vi "Compute Magnitudes.vi"(5 "view mode":enum16{"Power", "Amplitude", "dB"}(ring)=enum."Amplitude", 6 "averaging parameters":T1={"exponential mode"=enum."Fast", "time constant [ms]"=125.0, "decimating factor"=1} {"decimating factor" min=1 step=1; "time constant [ms]" format="%.2f"}, 7 "rpm range (auto)":T3 {"increment" format="%.2f"; "maximum" format="%.2f"; "minimum" format="%.2f"}, 9 "averaging type":enum16{"Linear", "Exponential"}(ring), 10 "speed profile":T4 {"speed [RPM]" format="%.2f"; "time [s]" format="%.2f"}, 11 "order waveforms [EU]":waveform(dbl)[](array[waveform])) -> (1 "unit label":string, 2 "magnitudes vs. rpm":T2(array[cluster]) {"magnitude" format="%.2f"; "delta rpm" format="%.2f"; "rpm 0" format="%.2f"}, 3 "orders magnitudes":waveform(dbl)[](array[waveform]))   [LabVIEW 2017]
doc: "Computes magnitudes for the order time waveforms."
uses:
  <vilib>/addons/Sound and Vibration/Order Analysis/Tach Process/SubVIs/speed profile.ctl
  <vilib>/addons/_NISVFA/_Shared subVIs/Common/svc_Engineering Units to Unit Label.vi
  <vilib>/addons/_NISVFA/_Shared subVIs/Common/svc_Unit Label to Engineering Units.vi
  <vilib>/Waveform/WDTOps.llb/WDT Index Channel DBL.vi
  <vilib>/addons/Sound and Vibration/Order Analysis/Gabor Order Tracking/SoundVib_Gabor.lvlib
  <vilib>/addons/Sound and Vibration/Order Analysis/Tach Process/SoundVib_TachProcess.lvlib
panel:
  # "Compute Magnitudes"
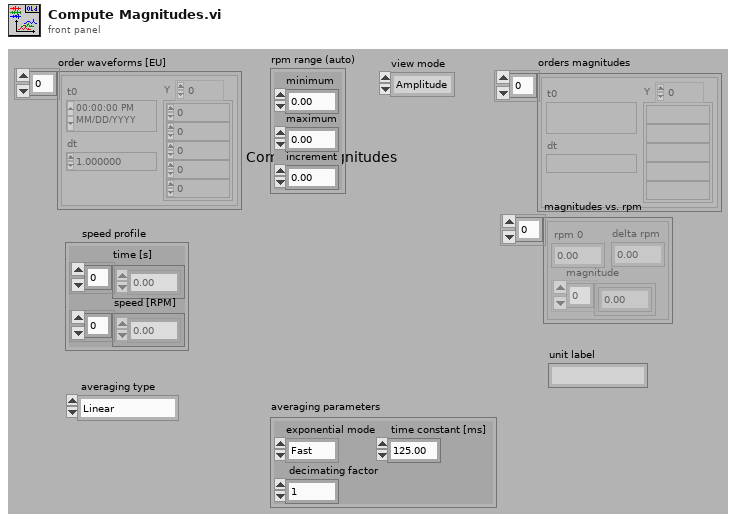
[diagram p1: front panel]
types:
  T1 = cluster{"exponential mode":enum16{"Slow", "Fast", "Impulse", "Custom"}, "time constant [ms]":dbl, "decimating factor":i32}
  T2 = cluster{"rpm 0":dbl, "delta rpm":dbl, "magnitude":dbl[]}[]
  T3 = cluster{"minimum":dbl, "maximum":dbl, "increment":dbl}
  T4 = typedef "SoundVib_TachProcess.lvlib/speed profile.ctl" = cluster{"time [s]":dbl[], "speed [RPM]":dbl[]}
  T5 = cluster{"Minimum":dbl, "Maximum":dbl, "Increment":dbl}
  T6 = typedef "svc_Channel Info.ctl" = cluster{"sensor sensitivity":dbl, "engineering units":T7, "dB reference":dbl, "custom label":string, "weighting filter":T8, "pregain":dbl}
  T7 = typedef "svc_Engineering Units Text Ring.ctl" = u16
  T8 = typedef "svc_Weighting Filter Text Ring.ctl" = u16
  T9 = cluster{"Minimum":dbl, "Increment":dbl, "log view scaled signal":dbl[]}
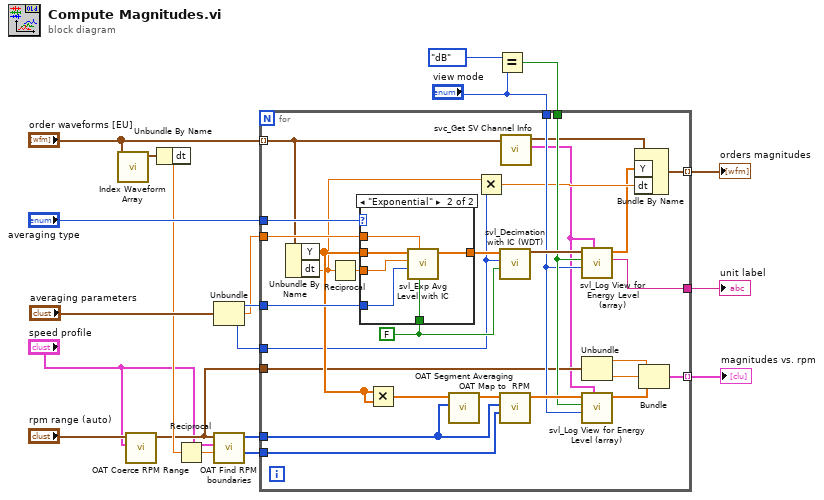
[diagram p0: block diagram]
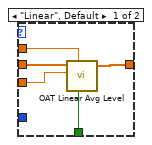
[diagram p2: hidden frame]
diagram:
  n1 = call-poly <vilib>:"Index Waveform Array.vi"("waveform array"="order waveforms [EU]") -> ("waveform"=w6:waveform(dbl))  [unwired: 9 in, 1 out]
  n2 = call <vilib>:"OAT Coerce RPM Range.vi"("speed profile"="speed profile", "RPM range in"="rpm range (auto)") -> ("RPM range out"=w4:T5)  [unwired: 3 in, 2 out]
  n3 = Unbundle By Name(w6) -> ("dt"=w5:dbl)
  n4 = Reciprocal(x=w5) -> (1/x=w2:dbl)
  n5 = Unbundle("averaging parameters") -> ("exponential mode"=w17:enum16{"Slow", "Fast", "Impulse", "Custom"}, "time constant [ms]"=w16:dbl, "decimating factor"=w8:i32)
  n6 = call <vilib>:"OAT Find RPM boundaries.vi"("sampling frequency [Hz]"=w2, "speed profile"="speed profile", "RPM range"=w4) -> ("RPM indices"=w14:i32[], "RPM boundaries"=w15:i32[])  [unwired: 3 in]
  n7 = Equal?(x=enum16{"Power", "Amplitude", "dB"}."dB" ("view mode"), y="view mode") -> (x = y?=w13:bool)
  n8 = for {
    tunnel: "order waveforms [EU]" -> [w23] mode=indexing
    tunnel: w17 -> [w49]
    tunnel: w16 -> [w48]
    tunnel: "averaging type" -> [w47]
    tunnel: w8 -> [w32]
    tunnel: w15 -> [w42]
    tunnel: w14 -> [w41]
    tunnel: w13 -> [w40]
    tunnel: "view mode" -> [w39]
    tunnel: [w38] -> w10
    tunnel: [w28] -> w9 mode=indexing
    tunnel: w4 -> [w27]
    tunnel: [w24] -> w3 mode=indexing
    w46 = FALSE ("init/cont (init:F)")
    n9 = Unbundle By Name(w23) -> ("Y"=w34:dbl[], "dt"=w31:dbl)
    n10 = Reciprocal(x=w31) -> (1/x=w33:dbl)
    n11 = case shown="\"Exponential\"" w47 {
      tunnel: w34 -> [w54 w60]
      tunnel: w33 -> [w53 w59]
      tunnel: w49 -> [_ w58]
      tunnel: w48 -> [w50 w57]
      tunnel: [w51 w56] -> w37
      tunnel: w46 -> [w52 w55]
      frame "Linear", Default {
        n12 = call <vilib>:"OAT Linear Avg Level.vi"("scaled signal [EU]"=w54, "time constant [ms]"=w50, "sampling frequency [Hz]"=w53, "init/cont (init:F)"=w52) -> ("linear avg level [EU^2 rms]"=w51:dbl[])  [unwired: 3 in, 1 out]
      }
      frame "Exponential" {
        n13 = call <vilib>:"svl_Exp Avg Level with IC.vi"("init/cont (init:F)"=w55, "time constant [ms]"=w57, "exponential mode"=w58, "sampling frequency [Hz]"=w59, "scaled signal [EU]"=w60) -> ("exp avg level [EU^2 rms]"=w56:dbl[])  [unwired: 4 in, 2 out]
      }
    }
    n14 = Multiply(x=w34, y=w34) -> (x*y=w36:dbl[])
    n15 = call <vilib>:"OAT Segment Averaging.vi"("boundaries"=w42, "Y [EU]"=w36) -> ("energy level in ranges [EU^2]"=w44:dbl[])  [unwired: 5 in]
    n16 = Multiply(x=w31, y=w32) -> (x*y=w30:dbl)
    n17 = call <vilib>:"svl_Decimation with IC (WDT).vi"("init/cont (init:F)"=w46, "decimating factor (1)"=w32, "expAveragedArray"=w37) -> ("expAveragedArray"=w45:waveform(dbl))  [unwired: 7 in, 1 out]
    n18 = call <vilib>:"OAT Map to  RPM.vi"("RPM indices"=w41, "RPM boundaries"=w42, "energy level in ranges"=w44) -> ("energy level at RPMs"=w43:dbl[])  [unwired: 4 in]
    n19 = call <vilib>:"svc_Get SV Channel Info.vi"("scaled signal [EU]"=w23) -> ("channel info"=w21:T6, "dup scaled signal [EU]"=w22:waveform(dbl))  [unwired: 5 in, 4 out]
    n20 = call <vilib>:"svl_Log View for Energy Level (array).vi"("channel info"=w21, "view mode"=w39, "dB On (T)"=w40, "scaled signal"=w45) -> ("unit label"=w38:string, "log view scaled signal"=w29:dbl[])  [unwired: 5 in, 1 out]
    n21 = Unbundle(w27) -> ("Minimum"=w26:dbl, "Increment"=w25:dbl)  [unwired: 1 out]
    n22 = call <vilib>:"svl_Log View for Energy Level (array).vi"("channel info"=w21, "view mode"=w39, "dB On (T)"=w40, "scaled signal"=w43) -> ("log view scaled signal"=w35:dbl[])  [unwired: 5 in, 2 out]
    n23 = Bundle By Name(cluster=w22, "Y"=w29, "dt"=w30) -> (w28:waveform(dbl))
    n24 = Bundle("Minimum"=w26, "Increment"=w25, "log view scaled signal"=w35) -> (w24:T9)  [unwired: 1 in]
  }
  "orders magnitudes" <- w9
  "magnitudes vs. rpm" <- w3
  "unit label" <- w10
